vi "Chilled water mixing valve PID.vi"(0 "Setpoint":dbl=15.0 format="%.2f", 1 "EnFlo_Tunnel:Chilled Water:Return":dbl, 2 "Previous Scan Value":dbl format="%.2f", 3 "Present Value":dbl=15.0 format="%.2f", 4 "Uni Chilled Water Temperature":dbl, 6 "Current Time":dbl) -> (5 "Dem Output":dbl format="%.2f")   [LabVIEW 2020]
uses:
  <vilib>/Analysis/NI_AALPro.lvlib
panel:
  out "Derivative":dbl(graph)
  out "Integral":dbl(graph)
  out "Proportional":dbl(graph)
  out "Error":dbl(graph)
  in  "Error DeadBand":dbl
  in  "O/P deadband":dbl=0.2 format="%.2f"
  in  "Kp Deadband":dbl format="%.2f"
  in  "Derivative History":i32=15
  out "deadbanded error":dbl format="%.2f"
  in  "P":bool=TRUE
  in  "D":bool=TRUE
  in  "I":bool=TRUE
  in  "Manual Demand":dbl min=0.0 max=100.0 format="%.2f"
  in  "Manual Override":bool
  out "PID Control Sum":dbl format="%.2f"
  out "error differential":dbl format="%.5f"
  in  "integral Term":dbl format="%.2f"
  in  "Kd":dbl=500.0 format="%.2f"
  in  "Ki":dbl=0.02 format="%.3f"
  in  "Kp":dbl=1.0 format="%.2f"
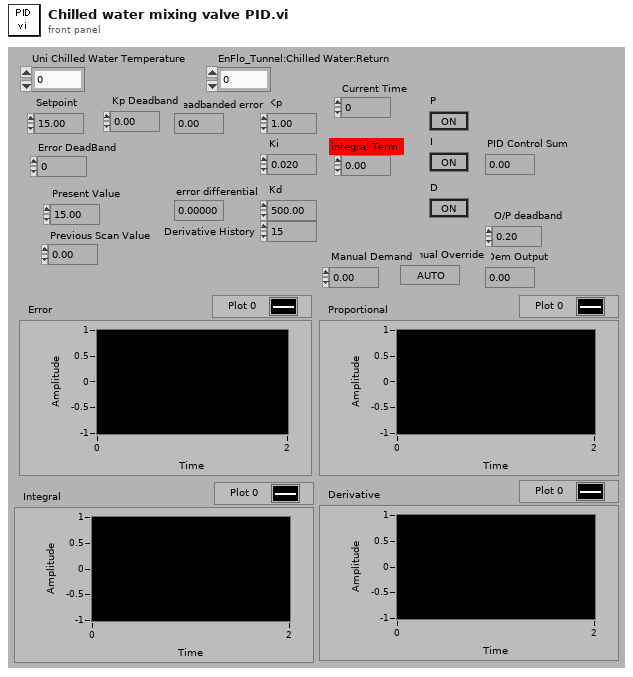
[diagram p1: front panel]
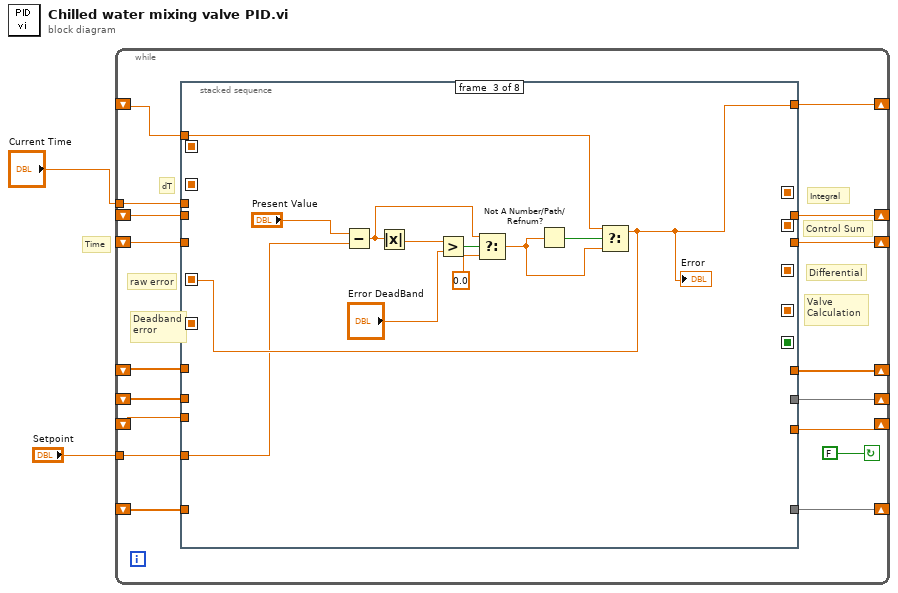
[diagram p0: block diagram]
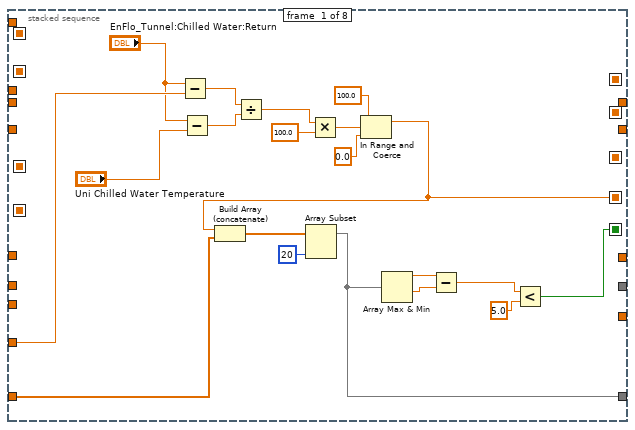
[diagram p2: hidden frame]
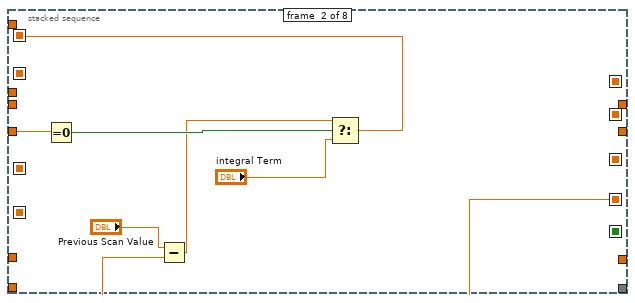
[diagram p3: hidden frame]
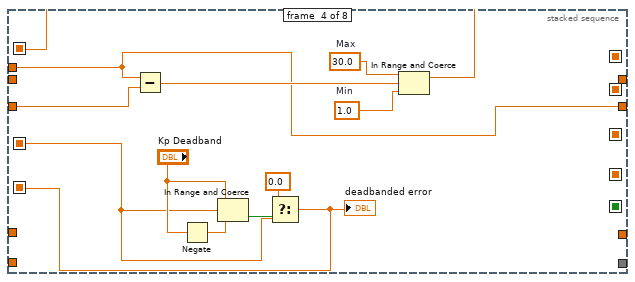
[diagram p4: hidden frame]
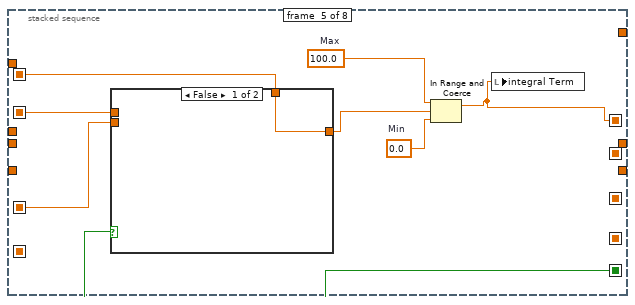
[diagram p5: hidden frame]
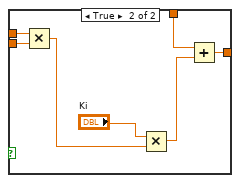
[diagram p6: hidden frame]
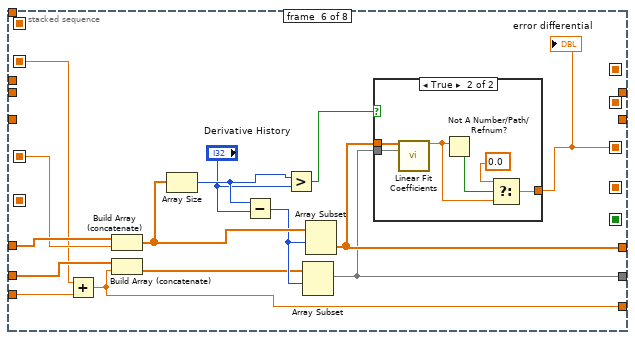
[diagram p7: hidden frame]
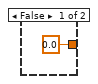
[diagram p8: hidden frame]
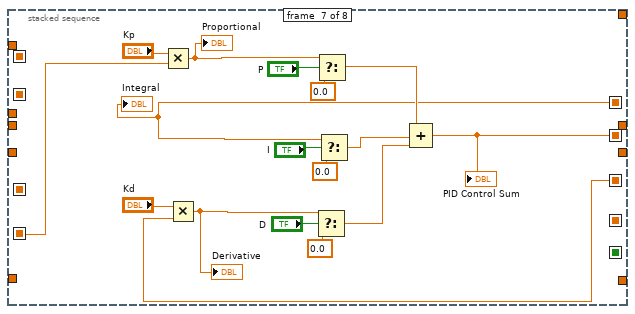
[diagram p9: hidden frame]
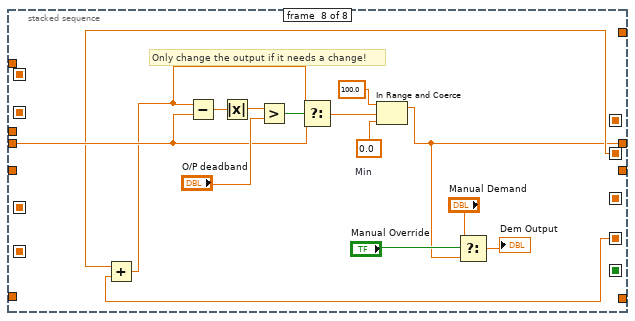
[diagram p10: hidden frame]
diagram:
  # "Time"
  n1 = while {
    shift-left: _ -> [w8]
    shift-right: [w7] -> _
    shift-left: _ -> [w10]
    shift-right: [w9] -> _
    shift-left: _ -> [w12]
    shift-right: [w11] -> _
    tunnel: "Current Time" -> [w17]
    shift-left: _ -> [w14]
    shift-right: [w13] -> _
    shift-left: _ -> [w16]
    shift-right: [w15] -> _
    shift-left: _ -> [w19]
    shift-right: [w18] -> _
    tunnel: "Setpoint" -> [w5]
    shift-right: [w4] -> _
    shift-left: _ -> [w3]
    stop <- FALSE continue-if-true
    # "Valve\nCalculation"
    # "Control Sum"
    # "raw error"
    # "Differential"
    # "Integral"
    # "Deadband\nerror"
    # "dT"
    n2 = stacked-sequence {
      seq-local: [_ _ _ w58 _ _ _ _] -> [_ _ _ _ w77 w91 _ _]
      seq-local: [_ _ _ w67 _ _ _ _] -> [_ _ _ _ _ _ w112 _]
      seq-local: [_ _ _ _ _ w93 _ _] -> [_ _ _ _ _ _ w111 _]
      seq-local: [_ _ _ _ w70 _ _ _] -> [_ _ _ _ _ _ w109 _]
      seq-local: [_ _ w48 _ _ _ _ _] -> [_ _ _ w59 w74 w94 _ _]
      seq-local: [_ _ _ _ _ _ w115 _] -> [_ _ _ _ _ _ _ w130]
      seq-local: [_ w44 _ _ _ _ _ _] -> [_ _ _ _ w72 _ _ _]
      seq-local: [w20 _ _ _ _ _ _ _] -> [_ w42 _ _ _ _ _ w131]
      seq-local: [w27 _ _ _ _ _ _ _] -> [_ _ _ _ w71 _ _ _]
      tunnel: w19 -> [_ w46 _ w64 _ _ _ _]
      tunnel: [_ _ _ w62 _ _ _ _] -> w18
      tunnel: w17 -> [_ _ _ w62 _ _ _ _]
      tunnel: w16 -> [_ _ _ _ _ w100 _ _]
      tunnel: [_ _ _ _ _ w95 _ _] -> w15
      tunnel: w14 -> [_ _ _ _ _ w99 _ _]
      tunnel: [_ _ _ _ _ w92 _ _] -> w13
      tunnel: w12 -> [_ _ _ _ _ _ _ w132]
      tunnel: [_ _ _ _ _ _ _ w125] -> w11
      tunnel: w10 -> [_ _ _ _ _ w90 _ _]
      tunnel: [_ _ _ _ _ w89 _ _] -> w9
      tunnel: w8 -> [_ _ w55 _ _ _ _ _]
      tunnel: [_ _ w48 _ _ _ _ _] -> w7
      tunnel: w5 -> [w26 _ w47 _ _ _ _ _]
      tunnel: [w31 _ _ _ _ _ _ _] -> w4
      tunnel: w3 -> [w32 _ _ _ _ _ _ _]
      frame #0 {
        n3 = Subtract(x="EnFlo_Tunnel:Chilled Water:Return", y=w26) -> (x-y=w39:dbl)
        n4 = Subtract(x="EnFlo_Tunnel:Chilled Water:Return", y="Uni Chilled Water Temperature") -> (x-y=w38:dbl)
        n5 = Divide(x=w39, y=w38) -> (x/y=w37:dbl)
        n6 = Multiply(x=w37, y=100.0) -> (x*y=w21:dbl)
        n7 = In Range and Coerce(upper limit=100.0, x=w21, lower limit=0.0) -> (coerced(x)=w20:dbl)  [unwired: 1 out]
        n8 = Build Array (concatenate)(w20, w32) -> (w34:dbl[])
        n9 = Array Subset(array=w34, length=20) -> (w31:dbl[])  [unwired: 1 in]
        n10 = Array Max & Min(array=w31) -> (max value=w30:dbl, min value=w29:dbl)  [unwired: 2 out]
        n11 = Subtract(x=w30, y=w29) -> (x-y=w28:dbl)
        n12 = Less?(x=w28, y=5.0) -> (x < y?=w27:bool)
      }
      frame #1 {
        n13 = Equal To 0?(x=w46) -> (x = 0?=w45:bool)
        n14 = Subtract(x="Previous Scan Value", y=w42) -> (x-y=w41:dbl)
        n15 = Select(t=w41, s=w45, f="integral Term") -> (s? t:f=w44:dbl)
      }
      frame #2 {
        n16 = Subtract(x="Present Value", y=w47) -> (x-y=w50:dbl)
        n17 = Absolute Value(x=w50) -> (abs(x)=w54:dbl)
        n18 = Greater?(x=w54, y="Error DeadBand") -> (0:w52:bool)
        n19 = Select(t=w50, s=w52, f=0.0 ("t")) -> (s? t:f=w51:dbl)
        n20 = Not A Number/Path/Refnum?(number/path/refnum=w51) -> (NaN/Path/Refnum?=w56:bool)
        n21 = Select(t=w55, s=w56, f=w51) -> (s? t:f=w48:dbl)
        "Error" <- w48
      }
      frame #3 {
        w65 = 1.0  # Min
        w66 = 30.0  # Max
        n22 = Subtract(x=w62, y=w64) -> (x-y=w63:dbl)
        n23 = Negate(x="Kp Deadband") -> (-x=w61:dbl)
        n24 = In Range and Coerce(upper limit="Kp Deadband", x=w59, lower limit=w61) -> (In Range?=w68:bool)  [unwired: 1 out]
        n25 = Select(t=0.0, s=w68, f=w59) -> (s? t:f=w67:dbl)
        "deadbanded error" <- w67
        n26 = In Range and Coerce(upper limit=w66, x=w63, lower limit=w65) -> (coerced(x)=w58:dbl)  [unwired: 1 out]
      }
      frame #4 {
        w76 = 0.0  # Min
        w73 = 100.0  # Max
        n27 = case shown="False" w71 {
          tunnel: w77 -> [_ w85]
          tunnel: [w78 w84] -> w75
          tunnel: w74 -> [_ w83]
          tunnel: w72 -> [w78 w79]
          frame False {
          }
          frame True {
            n28 = Multiply(x=w85, y=w83) -> (x*y=w81:dbl)
            n29 = Multiply(x="Ki", y=w81) -> (x*y=w82:dbl)
            n30 = Add(x=w79, y=w82) -> (x+y=w84:dbl)
          }
        }
        n31 = In Range and Coerce(upper limit=w73, x=w75, lower limit=w76) -> (coerced(x)=w70:dbl)  [unwired: 1 out]
        n32 = local write "integral Term"(w70) -> ()
      }
      frame #5 {
        n33 = Add(x=w91, y=w90) -> (x+y=w89:dbl)
        n34 = Build Array (concatenate)(w100, w94) -> (w98:dbl[])
        n35 = Build Array (concatenate)(w99, w89) -> (w96:dbl[])
        n36 = Array Size(array=w98) -> (size(s)=w87:i32)
        n37 = Subtract(x=w87, y="Derivative History") -> (x-y=w97:i32)
        n38 = Greater?(x=w87, y="Derivative History") -> (0:w88:bool)
        n39 = Array Subset(array=w96, index=w97) -> (w92:dbl[])  [unwired: 1 in]
        n40 = Array Subset(array=w98, index=w97) -> (w95:dbl[])  [unwired: 1 in]
        n41 = case shown="True" w88 {
          tunnel: w95 -> [_ w107]
          tunnel: [0.0 ("slope") w106] -> w93
          tunnel: w92 -> [_ w105]
          frame False {
          }
          frame True {
            n42 = call <vilib>:"Linear Fit Coefficients.vi"("Y"=w107, "X"=w105) -> ("slope"=w102:dbl)  [unwired: 3 in, 10 out]
            n43 = Not A Number/Path/Refnum?(number/path/refnum=w102) -> (NaN/Path/Refnum?=w104:bool)
            n44 = Select(t=0.0 ("f"), s=w104, f=w102) -> (s? t:f=w106:dbl)
          }
        }
        "error differential" <- w93
      }
      frame #6 {
        n45 = Multiply(x="Kp", y=w112) -> (x*y=w108:dbl)
        "Proportional" <- w108
        n46 = Multiply(x="Kd", y=w111) -> (x*y=w110:dbl)
        "Derivative" <- w110
        n47 = Select(t=w110, s="D", f=0.0) -> (s? t:f=w117:dbl)
        n48 = Select(t=w108, s="P", f=0.0) -> (s? t:f=w123:dbl)
        n49 = Select(t=w109, s="I", f=0.0) -> (s? t:f=w116:dbl)
        n50 = Compound Arithmetic op=ADD(w123, w116, w117) -> (w115:dbl)
        "PID Control Sum" <- w115
        "Integral" <- w109
      }
      frame #7 {
        w128 = 0.0  # Min
        # "Only change the output if it needs a change!"
        n51 = Add(x=w130, y=w131) -> (x+y=w129:dbl)
        n52 = Subtract(x=w129, y=w132) -> (x-y=w136:dbl)
        n53 = Absolute Value(x=w136) -> (abs(x)=w135:dbl)
        n54 = Greater?(x=w135, y="O/P deadband") -> (0:w134:bool)
        n55 = Select(t=w129, s=w134, f=w132) -> (s? t:f=w127:dbl)
        n56 = In Range and Coerce(upper limit=100.0, x=w127, lower limit=w128) -> (coerced(x)=w125:dbl)  [unwired: 1 out]
        n57 = Select(t="Manual Demand", s="Manual Override", f=w125) -> (s? t:f=→"Dem Output":dbl)
      }
    }
  }
